vi "Serialize.vi"(8 "error in (no error)":errorcluster, 11 "Job in":refnum<class "Job.lvclass">) -> (0 "error out":errorcluster, 2 "Text":string)   [LabVIEW 2014, in "Job.lvclass"]
uses:
  Job.lvclass
  Controls/Job Parameters - STYP.ctl
  Job.lvclass/Job.ctl
  Read Executor Number.vi
  Read WorkSpace Path.vi
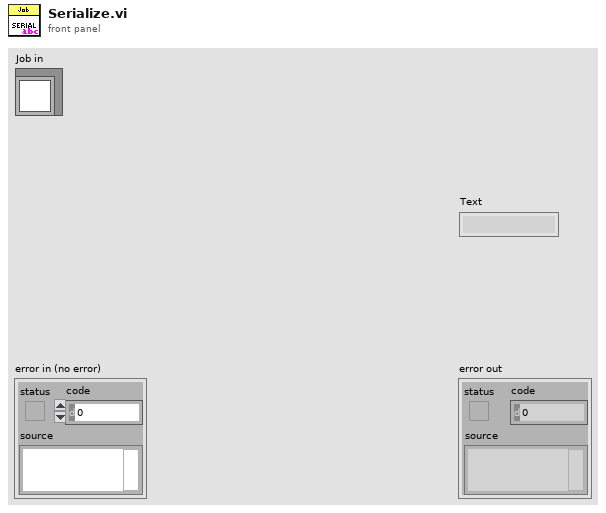
[diagram p1: front panel]
types:
  T1 = typedef "Job Parameters - STYP.ctl" = cluster{"Executor_Number":string, "Workspace_Path":string}
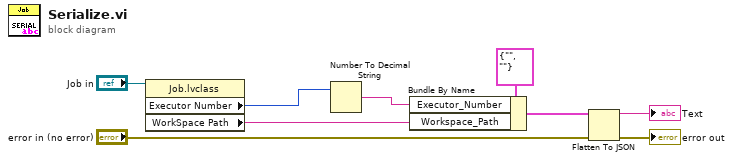
[diagram p0: block diagram]
diagram:
  n1 = property class="Job.lvclass"(reference="Job in") -> ("Executor Number"=w7:i32, "WorkSpace Path"=w8:string)  [unwired: 1 in, 2 out]
  n2 = Number To Decimal String(number=w7) -> (decimal integer string=w2:string)  [unwired: 1 in]
  n3 = Bundle By Name(cluster=T1 {"Executor_Number"="", "Workspace_Path"=""} ("Job_Param"), "Executor_Number"=w2, "Workspace_Path"=w8) -> (w9:T1)
  n4 = Flatten To JSON(anything=w9, error in (no error)="error in (no error)") -> (JSON string=→"Text":string, 11:→"error out":errorcluster)  [unwired: 1 in]
